vi "delay_ms.vi"(7 "delay(ms)":u32=100, 11 "错误输入（无错误）":errorcluster) -> (3 "错误输出":errorcluster)   [LabVIEW 2014]
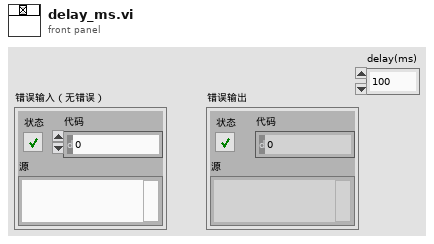
[diagram p1: front panel]
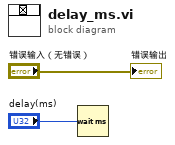
[diagram p0: block diagram]
diagram:
  n1 = Wait (ms)(milliseconds to wait="delay(ms)") -> ()  [unwired: 1 out]
  "错误输出" <- "错误输入（无错误）"
